vi "FuncImg-Event handler-Reinit controls.vi"(8 "error in":errorcluster, 9 "Number of POI":i32, 10 "Number of Miniscans":i32) -> (0 "Error out":errorcluster)   [LabVIEW 2020]
uses:
  Experiment header interface/Typedefs/Header file interface module functions enum.ctl
  Global variables/gl_Functional Imaging-Global variables.vi
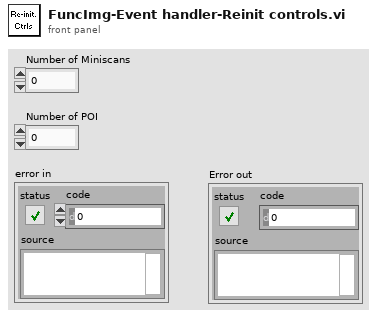
[diagram p1: front panel]
types:
  T1 = typedef "Header file interface module functions enum.ctl" = enum16{"Load experiment header file", "Save experiment header file", "Clear stored values", "Read stored values", "Update specific value in memory", "Update values in memory"}
  T2 = typedef "Functional Imging UI Refs.ctl" = cluster{"Menu ref":refnum<k9>, "Image control":refnum<vi>, "VI ref":refnum<vi>, "XGrapher":refnum<vi>, "Smoothing":refnum<vi>, "POI Averaging":refnum<vi>, "Normalize":refnum<vi>, "POI data points in each trial":refnum<vi>, "Channel":refnum<vi>, "Experiment data folder path":refnum<vi>, "[ROI vis]":refnum<vi>, "[Groups] visbl":T3, "Group Name":refnum<vi>, "POI index":refnum<vi>, "Trial No.":refnum<vi>, "Intensity Zoom":refnum<vi>, "Trial Cursor Enabled":refnum<vi>, "Number of Trials (ind 1)":refnum<vi>, "Number of Trials (ind 2)":refnum<vi>, "MiniScans Available":refnum<vi>, "POI Available":refnum<vi>, "Defer graph updates":refnum<vi>, "Waveform selector":refnum<vi>, "#of selected POI":refnum<vi>, "#of selected MiniScans":refnum<vi>, "#of selected groups":refnum<vi>, "Max Z-Projection":refnum<vi>, "Z-Plane Selector":refnum<vi>, "Index of miniscan point to visualise":refnum<vi>, "ROI vis. mode":refnum<vi>, "Total # of points":refnum<vi>, "Index of group clicked on":refnum<vi>, "Pane 1":refnum<vi>, "Pane 2":refnum<vi>, "Pane 3":refnum<vi>, "Pane 4":refnum<vi>, "Pane 5":refnum<vi>, "Pane 6":refnum<vi>, "Deselect all ROI":refnum<vi>, "Deselect all groups":refnum<vi>}
  T3 = typedef "Groups array referecne.ctl" = refnum<vi>
  T4 = typedef "Header parameters cluster-ALL.ctl" = cluster{"LOGIN":T5, "GLOBAL PARAMETERS":T6, "IMAGING MODES":T8, "TIME SERIES":T9, "MOTOR Z-STACK ":T12, "AOL Z-STACK":T13, "FUNCTIONAL IMAGING":T14, "VOLUME IMAGING":T14, "MOVEMENT CORRECTION":T18, "CALIBRATION":T20, "STATISTICS":T21, "BIOLOGY INFORMATION":T22, "Calibration Data":T23}
  T5 = typedef "Header params -Login.ctl" = cluster{"User":string, "Profile":string, "Software Version":string, "Experiment Date Time":timestamp}
  T6 = typedef "Header params-Global Parameters.ctl" = cluster{"MicroscopeID":string, "Microscope Type":string, "Objective":string, "Field of View (um)":dbl, "Fill time (us)":dbl, "Experiment Type":T7, "Stimuli Trigger":bool, "Speed Logging":bool}
  T7 = typedef "Experiment Type.ctl" = enum16{"In vivo", "In vitro", "Testing", "Calibration", "Other"}
  T8 = typedef "Header params-Imaging Modes.ctl" = cluster{"Time Series":bool, "Motor Zstack":bool, "AOL Zstack":bool, "Functional Imaging":bool, "Volume Imaging":bool}
  T9 = typedef "Header params-Time Series.ctl" = cluster{"Basic Image meta data":T10, "AOL z":dbl}
  T10 = typedef "Header params-Basic image meta data.ctl" = cluster{"Wavelength (nm)":dbl, "# averaged frames":dbl, "laser power (%)":dbl, "Pockels":dbl, "pixel dwell time (us)":dbl, "pmt 1":dbl, "pmt 2":dbl, "back apperture":dbl, "zoom":dbl, "field of view":dbl, "Frame Size":T11, "AOL x centre":dbl, "AOL y centre":dbl, "Stage x position":dbl, "Stage y position":dbl, "Stage z position":dbl}
  T11 = typedef "Frame Size.ctl" = u16
  T12 = typedef "Header params-Motor Z-stack.ctl" = cluster{"Hdr Basic Image meta data":T10, "Z Start":dbl, "Z Stop":dbl, "No of Planes":i32, "Laser Power (%) at Z Start":dbl, "Laser Power (%) at Z Stop":dbl}
  T13 = typedef "Header params-AOL Z-stack.ctl" = cluster{"Hdr Basic Image meta data":T10, "Z Start":dbl, "Z Stop":dbl, "No of Planes":i32, "Laser Power (%) at Z Start":dbl, "Laser Power (%) at Z Stop":dbl}
  T14 = typedef "Header params-Functional Imaging.ctl" = cluster{"Functional Mode":T15, "Variable Length":bool, "Variable Resolution":bool, "Pockels Modulation":bool, "Stimuli Trigger":bool, "Cool down enabled":bool, "AOL Mode":T16, "Plane Mode":T17, "Miniscan Dwell time per pixel (us)":dbl, "poi dwell time":dbl, "Number of trials":dbl, "Number of cycles":dbl, "Number of pois":dbl, "Number of miniscans":dbl, "Number of pixels in miniscan":dbl, "Rectangle ROI length":dbl, "Rectangle ROI height":dbl, "Frame rate (fps)":dbl, "Acquisition Length":dbl, "video length (sec)":dbl, "Stimuli delay (sec)":dbl, "Cool down time (sec)":dbl, "Basic Image meta data":T10, "Z Start (um)":dbl, "Z Stop (um)":dbl}
  T15 = typedef "Functional Mode.ctl" = enum16{"Point", "Line", "Patch", "Plane", "Volume"}
  T16 = typedef "AOL modes.ctl" = enum16{"Raster", "Structural", "Pointing", "Mini Scan", "Alignment"}
  T17 = typedef "Plane Mode.ctl" = u16
  T18 = typedef "Header params-Movement correction.ctl" = cluster{"Movement Correction":bool, "Axial Reference":bool, "Reference Source":T19, "Full Frame Size":dbl, "Reference Field of View":dbl, "Reference Zoom":dbl, "Reference dwell time (us)":dbl, "Reference X Pixels":dbl, "Reference Y Pixels":dbl, "Number of Z lines":dbl, "Size of Z pixels":dbl, "Axial Pixels":dbl, "Ignore Z lines":dbl, "Reference Scan Cycles":dbl, "Reference Threshold XY":dbl, "Reference Threshold Z":dbl, "Reference Average XY":dbl, "Reference Average Z":dbl, "Proportional Scale":dbl, "Integral Scale":dbl, "Proportional Scale Z":dbl, "Integral Scale Z":dbl, "Diff Threshold":dbl, "Diff Threshold Z":dbl, "Sliding Average":bool, "Reference count reset enabled":bool, "Scan Interval (ms)":dbl, "Ref Plot Refresh Rate (ms)":dbl}
  T19 = typedef "Reference source.ctl" = enum16{"Green channel", "Red channel"}
  T20 = typedef "Header params-Calibration Setup.ctl" = cluster{"Pockels Calibration File":path, "Calibration_ini file":path, "Setup_ini file":path}
  T21 = typedef "Header params-statistics.ctl" = cluster{"Z-stack duration (sec)":dbl, "Number of acquired data-points":dbl, "Acquisition time (ms)":dbl, "Number of acquired frames":dbl, "Intertrial times":dbl[]}
  T22 = typedef "Biology Information.ctl" = cluster{"Animal Code or Name":string, "Animal DoB":string, "Animal Age":string, "Animal Sex":string, "Animal Weight":string, "Date of Injection":string, "Date of Implant":string, "Site of Injection":string, "Animal Ear Notch":string, "AAV constructs":string, "Genetic background":string, "Optical reporter":string, "Region of brain imaged":string, "Other \ncomments":string}
  T23 = typedef "Header params-calibration data.ctl" = cluster{"Objective Name":string, "Calibration Wavelength":dbl, "Sum X":dbl, "Sum Y":dbl, "Diff X":dbl, "Diff Y":dbl, "Distortion Correction":dbl, " Z norm to um Scaling":dbl, " X norm to um Scaling":dbl}
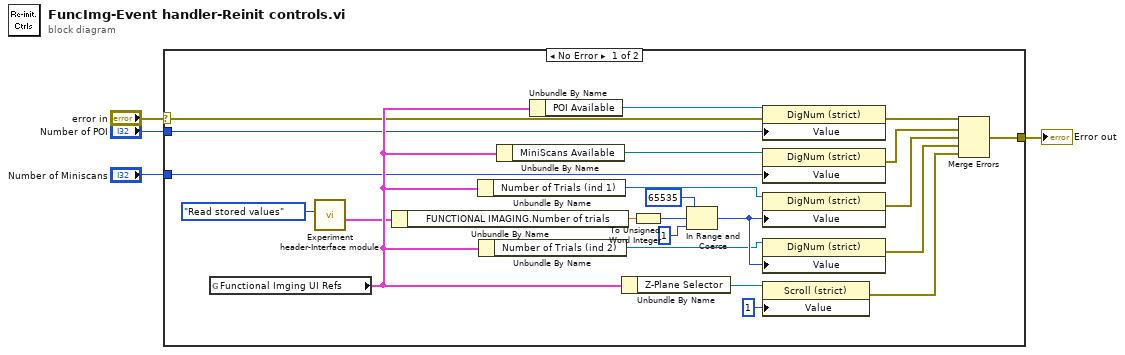
[diagram p0: block diagram]
diagram:
  n1 = case shown="No Error" "error in" {
    selector: "error in" -> [w15 w28]
    tunnel: "Number of Miniscans" -> [w20 _]
    tunnel: "Number of POI" -> [w19 _]
    tunnel: [w9 w28] -> w1
    frame No Error {
      n2 = global read "gl_Functional Imaging-Global variables.vi" "Functional Imging UI Refs"() -> (w27:T2)
      n3 = call "Experiment header-Interface module.vi"("Function"=Header_file_interface_module_functions_enum."Read stored values") -> ("All header parameters out"=w7:T4)  [unwired: 9 in, 1 out]
      n4 = Unbundle By Name(w7) -> ("FUNCTIONAL IMAGING.Number of trials"=w5:dbl)
      n5 = Unbundle By Name(w27) -> ("Number of Trials (ind 1)"=w16:refnum<vi>)
      n6 = Unbundle By Name(w27) -> ("Number of Trials (ind 2)"=w17:refnum<vi>)
      n7 = Unbundle By Name(w27) -> ("MiniScans Available"=w21:refnum<vi>)
      n8 = Unbundle By Name(w27) -> ("POI Available"=w18:refnum<vi>)
      n9 = Unbundle By Name(w27) -> ("Z-Plane Selector"=w26:refnum<vi>)
      n10 = To Unsigned Word Integer(number=w5) -> (unsigned 16bit integer=w6:u16)
      n11 = In Range and Coerce(upper limit=u16 65535, x=w6, lower limit=u16 1) -> (coerced(x)=w22:u16)  [unwired: 1 out]
      n12 = property on="Property Node" class="DigNum (strict)"(reference=w18, error in=w15, "Value"=w19) -> (error out=w14:errorcluster)  [unwired: 1 out]
      n13 = property on="Property Node" class="DigNum (strict)"(reference=w21, "Value"=w20) -> (error out=w13:errorcluster)  [unwired: 1 in, 1 out]
      n14 = property on="Property Node" class="DigNum (strict)"(reference=w16, "Value"=w22) -> (error out=w12:errorcluster)  [unwired: 1 in, 1 out]
      n15 = property on="Property Node" class="DigNum (strict)"(reference=w17, "Value"=w22) -> (error out=w11:errorcluster)  [unwired: 1 in, 1 out]
      n16 = property on="Property Node" class="Scroll (strict)"(reference=w26, "Value"=1) -> (error out=w10:errorcluster)  [unwired: 1 in, 1 out]
      n17 = Merge Errors(w14, w13, w12, w11, w10) -> (w9:errorcluster)
    }
    frame Error {
    }
  }
  "Error out" <- w1
